vi "WriteConfig.vi"() -> ()   [LabVIEW 2022 SP3]
uses:
  TopLevel/Typedefs/Digilens Config Cluster.ctl
  TopLevel/Typedefs/Motor Controller Config Data.ctl
  IO/Typedefs/IO Config Data.ctl
  IO/Typedefs/DCON_DeviceConfig--Cluster.ctl
  IO/Typedefs/Channel Data.ctl
  GIS Printer/Typedefs/PrinterConfiguration--Cluster.ctl
  DAQWFE/LV_Source/Subsystems/DAQ/DataTypes/TD DAQ Settings--cluster.ctl
  DAQWFE/LV_Source/Subsystems/DAQ/DataTypes/TD DI Instrument Settings--cluster.ctl
  DAQWFE/LV_Source/Subsystems/DAQ/DataTypes/TD AI Instrument Settings--cluster.ctl
  DAQWFE/LV_Source/Subsystems/DAQ/DataTypes/TD AI InstSettings--cluster.ctl
  DAQWFE/LV_Source/Subsystems/DAQ/Process/ProcessSupport/TD SimAI Ranges--cluster.ctl
  Motor Controller/Motor Controller.lvclass
  TopLevel/TopLevel.lvclass
  IO/IO.lvclass
  GIS Printer/GIS Printer.lvclass
  DAQWFE/LV_Source/Subsystems/DAQ/DAQ.lvclass
panel:
  in  "XML File Path":path=path "C:/projects/Digilens_IPLC/MasterConfiguration.xml"
  in  "Digilens IPLC Config":T1={"Motion Controller"={"Motor IP Addresss"="192.168.1.12", "Current Position"=2, "Pulse_Per_mm"=100, "PrePrint"=[], "Load Position_mm"=0, "Laminate Position_mm"=2}, "IO Config"={"DAQDevices"=[{"COM"="COM12", "DeviceName"="ICP2-DI", "BaudRate"=115200, "Number of Channels"=16, "DeviceAddress"=2, "Enable"=TRUE}, {"COM"="COM12", "DeviceName"="ICP2-DO", "BaudRate"=115200, "Number of Channels"=32, "DeviceAddress"=3, "Enable"=TRUE}, {"COM"="COM12", "DeviceName"="ICP1-DO", "BaudRate"=115200, "Number of Channels"=0, "DeviceAddress"=0, "Enable"=FALSE}, {"COM"="COM10", "DeviceName"="ICP1-AI", "BaudRate"=115600, "Number of Channels"=8, "DeviceAddress"=2, "Enable"=TRUE}, {"COM"="COM10", "DeviceName"="ICP1-AO", "BaudRate"=115200, "Number of Channels"=8, "DeviceAddress"=3, "Enable"=TRUE}, {"COM"="COM12", "DeviceName"="ICP2-AO", "BaudRate"=115200, "Number of Channels"=8, "DeviceAddress"=4, "Enable"=TRUE}], "DI Channels"=[{"Channel Name"="SW - Ink Valve - R1", "Device Name"="ICP2-DI", "Channel No"="16"}, {"Channel Name"="SW - Ink Valve - R2", "Device Name"="ICP2-DI", "Channel No"="1"}, {"Channel Name"="SW - Ink Valve - R3", "Device Name"="ICP2-DI", "Channel No"="2"}, {"Channel Name"="SW - Ink Valve - R4", "Device Name"="ICP2-DI", "Channel No"="3"}, {"Channel Name"="SW - Ink Valve - R5", "Device Name"="ICP2-DI", "Channel No"="4"}, {"Channel Name"="SW - Ink Valve - R6", "Device Name"="ICP2-DI", "Channel No"="5"}, {"Channel Name"="SW - COVER INPUT SIDE", "Device Name"="ICP2-DI", "Channel No"="6"}, {"Channel Name"="SW - COVER OUTPUT SIDE", "Device Name"="ICP2-DI", "Channel No"="7"}, {"Channel Name"="SW - Purge - R1", "Device Name"="ICP2-DI", "Channel No"="10"}, {"Channel Name"="SW - Purge - R2", "Device Name"="ICP2-DI", "Channel No"="11"}, {"Channel Name"="SW - Purge - R3", "Device Name"="ICP2-DI", "Channel No"="12"}, {"Channel Name"="SW - Purge - R4", "Device Name"="ICP2-DI", "Channel No"="13"}, {"Channel Name"="SW - Purge - R5", "Device Name"="ICP2-DI", "Channel No"="14"}, {"Channel Name"="SW - Purge - R6", "Device Name"="ICP2-DI", "Channel No"="15"}], "DO Channels"=[{"Channel Name"="Meniscus Pressure Reg PWR - R1", "Device Name"="ICP1-DO", "Channel No"="0"}, {"Channel Name"="Meniscus Pressure Reg PWR - R2", "Device Name"="ICP1-DO", "Channel No"="1"}, {"Channel Name"="Meniscus Pressure Reg PWR - R3", "Device Name"="ICP1-DO", "Channel No"="2"}, {"Channel Name"="Meniscus Pressure Reg PWR - R4", "Device Name"="ICP1-DO", "Channel No"="3"}, {"Channel Name"="Meniscus Pressure Reg PWR - R5", "Device Name"="ICP1-DO", "Channel No"="4"}, {"Channel Name"="Meniscus Pressure Reg PWR - R6", "Device Name"="ICP1-DO", "Channel No"="5"}, {"Channel Name"="Purge Valve Open - R1", "Device Name"="ICP1-DO", "Channel No"="10"}, {"Channel Name"="Purge Valve Open - R2", "Device Name"="ICP1-DO", "Channel No"="11"}, {"Channel Name"="Purge Valve Open - R3", "Device Name"="ICP1-DO", "Channel No"="12"}, {"Channel Name"="Purge Valve Open - R4", "Device Name"="ICP1-DO", "Channel No"="13"}, {"Channel Name"="Purge Valve Open - R5", "Device Name"="ICP1-DO", "Channel No"="14"}, {"Channel Name"="Purge Valve Open - R6", "Device Name"="ICP1-DO", "Channel No"="15"}, {"Channel Name"="Meniscus Valve Open - R1", "Device Name"="ICP2-DO", "Channel No"="0"}, {"Channel Name"="Meniscus Valve Open - R2", "Device Name"="ICP2-DO", "Channel No"="1"}, {"Channel Name"="Meniscus Valve Open - R3", "Device Name"="ICP2-DO", "Channel No"="2"}, {"Channel Name"="Meniscus Valve Open - R4", "Device Name"="ICP2-DO", "Channel No"="3"}, {"Channel Name"="Meniscus Valve Open - R5", "Device Name"="ICP2-DO", "Channel No"="4"}, {"Channel Name"="Meniscus Valve Open - R6", "Device Name"="ICP2-DO", "Channel No"="5"}, {"Channel Name"="Ink Flow Valve Open - R1", "Device Name"="ICP2-DO", "Channel No"="10"}, {"Channel Name"="Ink Flow Valve Open - R2", "Device Name"="ICP2-DO", "Channel No"="11"}, {"Channel Name"="Ink Flow Valve Open - R3", "Device Name"="ICP2-DO", "Channel No"="12"}, {"Channel Name"="Ink Flow Valve Open - R4", "Device Name"="ICP2-DO", "Channel No"="13"}, {"Channel Name"="Ink Flow Valve Open - R5", "Device Name"="ICP2-DO", "Channel No"="14"}, {"Channel Name"="Ink Flow Valve Open - R6", "Device Name"="ICP2-DO", "Channel No"="15"}, {"Channel Name"="SW_LED - Ink Valve - R1", "Device Name"="ICP2-DO", "Channel No"="16"}, {"Channel Name"="SW_LED - Ink Valve - R2", "Device Name"="ICP2-DO", "Channel No"="17"}, {"Channel Name"="SW_LED - Ink Valve - R3", "Device Name"="ICP2-DO", "Channel No"="18"}, {"Channel Name"="Recirc Pump On - R1", "Device Name"="ICP2-DO", "Channel No"="20"}, {"Channel Name"="Recirc Pump On - R2", "Device Name"="ICP2-DO", "Channel No"="21"}, {"Channel Name"="Recirc Pump On - R3", "Device Name"="ICP2-DO", "Channel No"="22"}, {"Channel Name"="Recirc Pump On - R4", "Device Name"="ICP2-DO", "Channel No"="23"}, {"Channel Name"="Recirc Pump On - R5", "Device Name"="ICP2-DO", "Channel No"="24"}, {"Channel Name"="Recirc Pump On - R6", "Device Name"="ICP2-DO", "Channel No"="25"}, {"Channel Name"="SW_LED - Ink Valve - R4", "Device Name"="ICP2-DO", "Channel No"="26"}, {"Channel Name"="SW_LED - Ink Valve - R5", "Device Name"="ICP2-DO", "Channel No"="27"}, {"Channel Name"="SW_LED - Ink Valve - R6", "Device Name"="ICP2-DO", "Channel No"="28"}], "Material Names"=["none", "113A.3", "507.2-1", "109G"], "AI Channels"=[{"Channel Name"="Meniscus Pressure Read - R1", "Device Name"="ICP1-AI", "Channel No"="0"}, {"Channel Name"="Meniscus Pressure Read - R2", "Device Name"="ICP1-AI", "Channel No"="1"}, {"Channel Name"="Meniscus Pressure Read - R3", "Device Name"="ICP1-AI", "Channel No"="2"}, {"Channel Name"="Meniscus Pressure Read - R4", "Device Name"="ICP1-AI", "Channel No"="3"}, {"Channel Name"="Meniscus Pressure Read - R5", "Device Name"="ICP1-AI", "Channel No"="4"}, {"Channel Name"="Meniscus Pressure Read - R6", "Device Name"="ICP1-AI", "Channel No"="5"}], "AO Channels"=[{"Channel Name"="Meniscus Pressure Set - R1", "Device Name"="ICP1-AO", "Channel No"="0"}, {"Channel Name"="Meniscus Pressure Set - R2", "Device Name"="ICP1-AO", "Channel No"="1"}, {"Channel Name"="Meniscus Pressure Set - R3", "Device Name"="ICP1-AO", "Channel No"="2"}, {"Channel Name"="Meniscus Pressure Set - R4", "Device Name"="ICP1-AO", "Channel No"="3"}, {"Channel Name"="Meniscus Pressure Set - R5", "Device Name"="ICP1-AO", "Channel No"="4"}, {"Channel Name"="Meniscus Pressure Set - R6", "Device Name"="ICP1-AO", "Channel No"="5"}, {"Channel Name"="Recirc Pump Flow Set - R1", "Device Name"="ICP2-AO", "Channel No"="0"}, {"Channel Name"="Recirc Pump Flow Set - R2", "Device Name"="ICP2-AO", "Channel No"="1"}, {"Channel Name"="Recirc Pump Flow Set - R3", "Device Name"="ICP2-AO", "Channel No"="2"}, {"Channel Name"="Recirc Pump Flow Set - R4", "Device Name"="ICP2-AO", "Channel No"="3"}, {"Channel Name"="Recirc Pump Flow Set - R5", "Device Name"="ICP2-AO", "Channel No"="4"}, {"Channel Name"="Recirc Pump Flow Set - R6", "Device Name"="ICP2-AO", "Channel No"="5"}]}, "PrinterConfiguration"={"IPAddress"="localhost", "Move Stage on RTP Command?"=TRUE, "Stage Move Position"="Laminate", "PH1-Prime Path"=path "C:/projects/Digilens_IPLC/Scripts/PH1-PRIME.txt", "PH2-Prime Path"=path "C:/projects/Digilens_IPLC/Scripts/PH2-PRIME.txt", "PH3-Prime Path"=path "C:/projects/Digilens_IPLC/Scripts/PH3-PRIME.txt", "PH4-Prime Path"=path "C:/projects/Digilens_IPLC/Scripts/PH4-PRIME.txt", "PH5-Prime Path"=path "C:/projects/Digilens_IPLC/Scripts/PH5-PRIME.txt", "PH6-Prime Path"=path "C:/projects/Digilens_IPLC/Scripts/PH6-PRIME.txt", "PrintScriptsFolder"=path "", "PurgeScriptsFolder"=path "", "StageScriptsFolder"=path "", "PH1-HeatOn Path"=path "", "PH2-HeatOn Path"=path "", "PH3-HeatOn Path"=path "", "PH4-HeatOn Path"=path "", "PH5-HeatOn Path"=path "", "PH6-HeatOn Path"=path "", "PH1-HeatOff Path"=path "", "PH2-HeatOff Path"=path "", "PH3-HeatOff Path"=path "", "PH4-HeatOff Path"=path "", "PH5-HeatOff Path"=path "", "PH6-HeatOff Path"=path ""}, "DAQ Settings"={"Simulate DAQ"=FALSE, "DI Settings"=[{"Disable"=FALSE, "DI TaskName"="DITask_1", "DI RefreshIntv"=10}], "AI Settings"=[{"Disable"=FALSE, "AI TaskName"="AITask_1", "AI InstSettings"={"DaqRate"=100.0, "NumSamples"=1}, "SimAI Ranges"={"lo"=4.0, "hi"=20.0}}], "Relay IONames"=["Meniscus Pressure Reg PWR - R1", "Meniscus Pressure Reg PWR - R2", "Meniscus Pressure Reg PWR - R3", "Meniscus Pressure Reg PWR - R4", "Meniscus Pressure Reg PWR - R5", "Meniscus Pressure Reg PWR - R6", "SV2 Servo Enable", "SV2 Servo ON", "Purge Valve Open - R1", "Purge Valve Open - R2", "Purge Valve Open - R3", "Purge Valve Open - R4", "Purge Valve Open - R5", "Purge Valve Open - R6", "Meniscus Valve Open - R1", "Meniscus Valve Open - R2", "Meniscus Valve Open - R3", "Meniscus Valve Open - R4", "Meniscus Valve Open - R5", "Meniscus Valve Open - R6", "Ink Flow Valve Open - R1", "Ink Flow Valve Open - R2", "Ink Flow Valve Open - R3", "Ink Flow Valve Open - R4", "Ink Flow Valve Open - R5", "Ink Flow Valve Open - R6", "Recirc Pump On - R1", "Recirc Pump On - R2", "Recirc Pump On - R3", "Recirc Pump On - R4", "Recirc Pump On - R5", "Recirc Pump On - R6", "LED - Ink Valve Switch - R1", "LED - Ink Valve Switch - R2", "LED - Ink Valve Switch - R3", "LED - Ink Valve Switch - R4", "LED - Ink Valve Switch - R5", "LED - Ink Valve Switch - R6"], "AO IONames"=["Meniscus Pressure Set - R1", "Meniscus Pressure Set - R2", "Meniscus Pressure Set - R3", "Meniscus Pressure Set - R4", "Meniscus Pressure Set - R5", "Meniscus Pressure Set - R6"], "AO NChan SingleTask"=FALSE}}
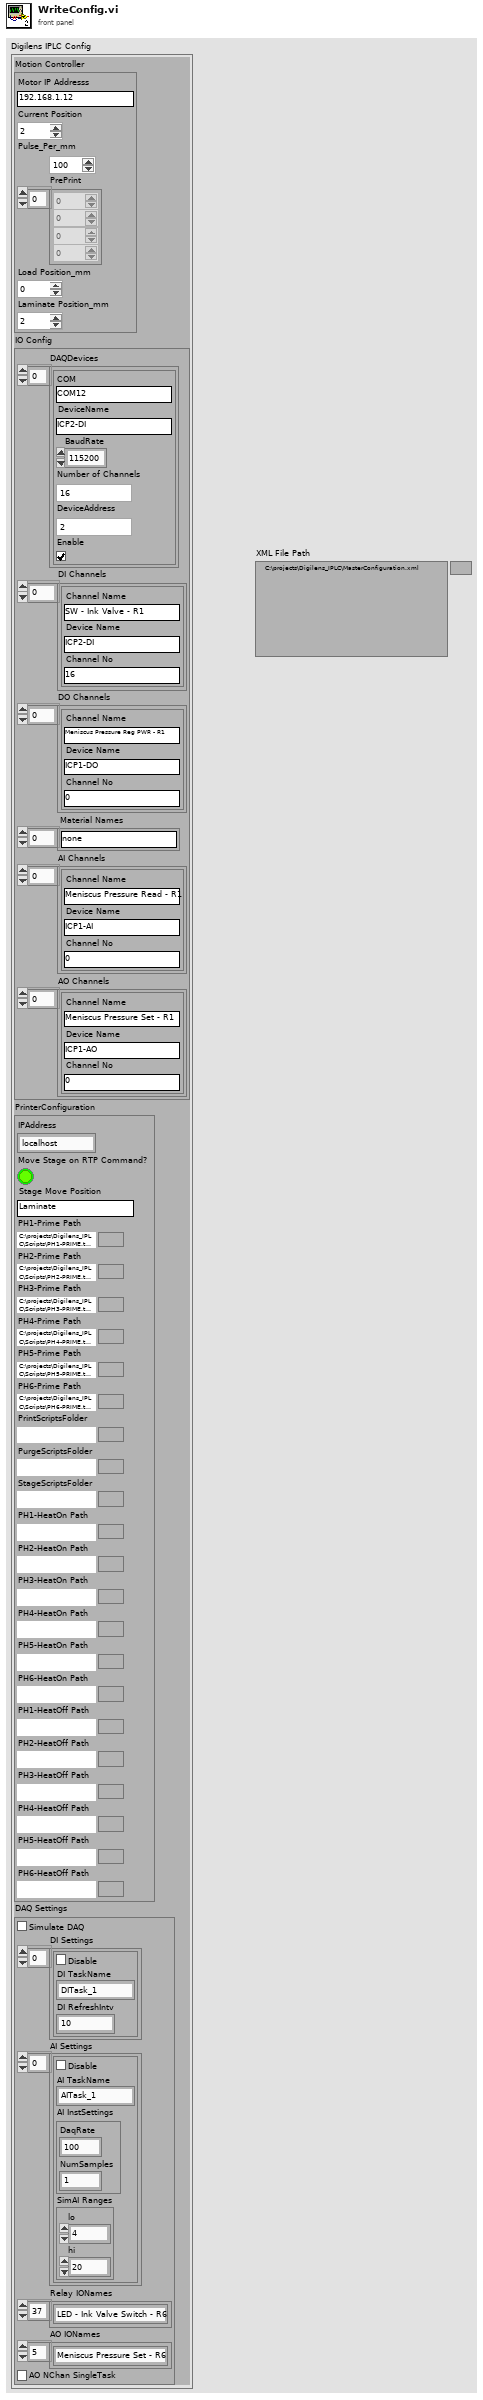
[diagram p1: front panel]
types:
  T1 = typedef "TopLevel.lvclass/Digilens Config Cluster.ctl" = cluster{"Motion Controller":T2, "IO Config":T3, "PrinterConfiguration":T6, "DAQ Settings":T7}
  T2 = typedef "Motor Controller.lvclass/Motor Controller Config Data.ctl" = cluster{"Motor IP Addresss":string, "Current Position":i32, "Pulse_Per_mm":i32, "PrePrint":dbl[], "Load Position_mm":i32, "Laminate Position_mm":i32}
  T3 = typedef "IO.lvclass/IO Config Data.ctl" = cluster{"DAQDevices":T4[], "DI Channels":T5[], "DO Channels":T5[], "Material Names":string[], "AI Channels":T5[], "AO Channels":T5[]}
  T4 = typedef "IO.lvclass/DCON_DeviceConfig--Cluster.ctl" = cluster{"COM":string, "DeviceName":string, "BaudRate":u32, "Number of Channels":i32, "DeviceAddress":i32, "Enable":bool}
  T5 = typedef "IO.lvclass/Channel Data.ctl" = cluster{"Channel Name":string, "Device Name":string, "Channel No":string}
  T6 = typedef "GIS Printer.lvclass/PrinterConfiguration--Cluster.ctl" = cluster{"IPAddress":string, "Move Stage on RTP Command?":bool, "Stage Move Position":string, "PH1-Prime Path":path, "PH2-Prime Path":path, "PH3-Prime Path":path, "PH4-Prime Path":path, "PH5-Prime Path":path, "PH6-Prime Path":path, "PrintScriptsFolder":path, "PurgeScriptsFolder":path, "StageScriptsFolder":path, "PH1-HeatOn Path":path, "PH2-HeatOn Path":path, "PH3-HeatOn Path":path, "PH4-HeatOn Path":path, "PH5-HeatOn Path":path, "PH6-HeatOn Path":path, "PH1-HeatOff Path":path, "PH2-HeatOff Path":path, "PH3-HeatOff Path":path, "PH4-HeatOff Path":path, "PH5-HeatOff Path":path, "PH6-HeatOff Path":path}
  T7 = typedef "DAQ.lvclass/TD DAQ Settings--cluster.ctl" = cluster{"Simulate DAQ":bool, "DI Settings":T8[], "AI Settings":T9[], "Relay IONames":string[], "AO IONames":string[], "AO NChan SingleTask":bool}
  T8 = typedef "DAQ.lvclass/TD DI Instrument Settings--cluster.ctl" = cluster{"Disable":bool, "DI TaskName":string, "DI RefreshIntv":i32}
  T9 = typedef "DAQ.lvclass/TD AI Instrument Settings--cluster.ctl" = cluster{"Disable":bool, "AI TaskName":string, "AI InstSettings":T10, "SimAI Ranges":T11}
  T10 = typedef "DAQ.lvclass/TD AI InstSettings--cluster.ctl" = cluster{"DaqRate":dbl, "NumSamples":i32}
  T11 = typedef "DAQ.lvclass/TD SimAI Ranges--cluster.ctl" = cluster{"lo":dbl, "hi":dbl}
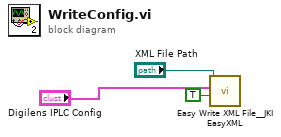
[diagram p0: block diagram]
diagram:
  n1 = call <vilib>:"Easy Write XML File__JKI EasyXML.vi"("Overwrite File? (false)"=TRUE, "LabVIEW Data"="Digilens IPLC Config", "XML File Path"="XML File Path") -> ()  [unwired: 7 in, 2 out]
